vi "WriteTraceQueue.vi"(8 "Error In":errorcluster, 10 "TraceQueue":refnum<queue>, 11 "reference in":refnum<class "TraceWindow.lvclass">) -> (0 "Error Out":errorcluster, 3 "reference in":refnum<class "TraceWindow.lvclass">)   [LabVIEW 2021, in "TraceWindow.lvlib" / "TraceWindow.lvclass"]
uses:
  TraceWindow.lvclass
  protected/TraceWindow_MessageData.ctl
  26c62d72-41ba-42b8-a08f-c4964286269c.vi
  protected/MainGUIRepository.vi
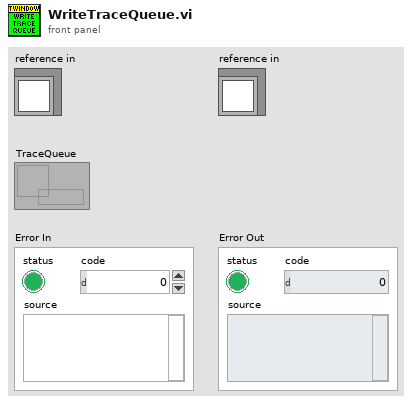
[diagram p1: front panel]
types:
  T1 = typedef "TraceWindow.lvlib/TraceWindow.lvclass/TraceWindow_MessageData.ctl" = cluster{"Show":cluster{"Send":cluster{"State":bool}, "Receive":cluster{"Dummy":bool}}, "WriteTraceQueue":cluster{"Send":cluster{"TraceQueue":refnum<queue>}, "Receive":cluster{"Dummy":bool}}}
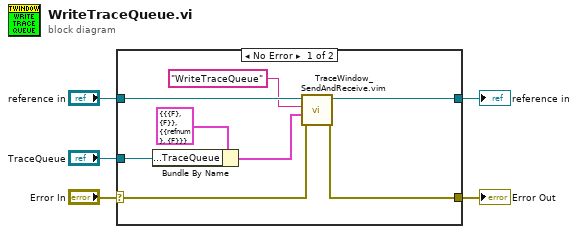
[diagram p0: block diagram]
diagram:
  n1 = case shown="No Error" "Error In" {
    selector: "Error In" -> [w11 w15]
    tunnel: [w10 w15] -> w4
    tunnel: [w12 w14] -> w2
    tunnel: "reference in" -> [w13 w14]
    tunnel: "TraceQueue" -> [w8 _]
    frame No Error {
      n2 = Bundle By Name(cluster=T1 {"Show"={"Send"={"State"=FALSE}, "Receive"={"Dummy"=FALSE}}, "WriteTraceQueue"={"Send"={"TraceQueue"=refnum}, "Receive"={"Dummy"=FALSE}}} ("MessageData"), "WriteTraceQueue.Send.TraceQueue"=w8) -> (w7:T1)
      n3 = call "TraceWindow_SendAndReceive.vim"("error in (no error)"=w11, "Data"=w7, "Command"="WriteTraceQueue", "reference in"=w13) -> ("error out"=w10:errorcluster, "reference out"=w12:refnum<class "TraceWindow.lvclass">)  [unwired: 5 in, 1 out]
    }
    frame Error {
    }
  }
  "Error Out" <- w4
  "reference in" <- w2
